vi "Reset Redlines.vi"(8 "error in (no error)":errorcluster, 11 "BluelinesRedlines in":refnum<class "BluelinesRedlines.lvclass">) -> (0 "error out":errorcluster, 3 "BluelinesRedlines out":refnum<class "BluelinesRedlines.lvclass">)   [LabVIEW 2020, in "VolatusGUIElements.lvlib" / "BluelinesRedlines.lvclass"]
uses:
  BluelinesRedlines.lvclass
  BluelinesRedlines.lvclass/BluelinesRedlines.ctl
  VolatusGUI/BluelinesRedlines Source/BluelinesRedlines Source.lvclass
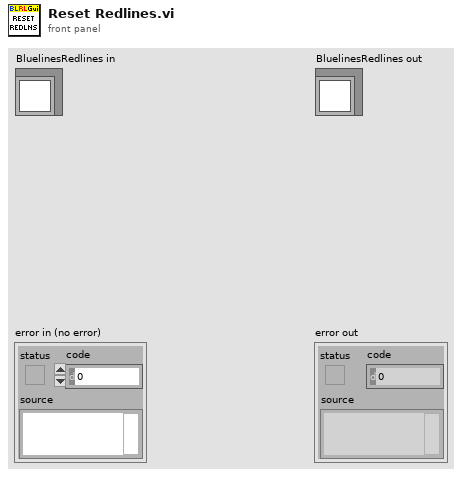
[diagram p1: front panel]
types:
  T1 = map{string, refnum<class "BluelinesRedlines Source.lvclass">}
  T2 = typedef "VolatusGUI.lvlib/BluelinesRedlines Source.lvclass/BLRL Config.ctl" = cluster{"Bluelines":T3[], "Redlines":T3[]}
  T3 = typedef "VolatusGUI.lvlib/BluelinesRedlines Source.lvclass/Range Limit Config.ctl" = cluster{"Channel":string, "Low Limit":dbl, "High Limit":dbl}
  T4 = typedef "VolatusGUIElements.lvlib/BluelinesRedlines.lvclass/Channel Info.ctl" = cluster{"Channel":refnum<class "Channel DBL.lvclass">, "Redline":bool}
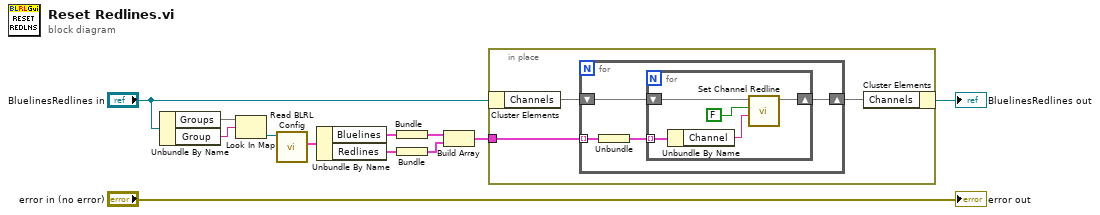
[diagram p0: block diagram]
diagram:
  n1 = Unbundle By Name("BluelinesRedlines in") -> ("Groups"=w4:T1, "Group"=w3:string)
  n2 = Look In Map(map=w4, key=w3) -> (value=w10:refnum<class "BluelinesRedlines Source.lvclass">)  [unwired: 1 in, 1 out]
  n3 = call-dynamic "Read BLRL Config.vi"("BluelinesRedlines Source in"=w10) -> ("BLRL Config"=w5:T2)  [unwired: 8 in, 2 out]
  n4 = Unbundle By Name(w5) -> ("Bluelines"=w9:T3[], "Redlines"=w8:T3[])
  n5 = Bundle("Bluelines"=w9) -> (w7:cluster{"Bluelines":T3[]})  [unwired: 1 in]
  n6 = Bundle("Redlines"=w8) -> (w6:cluster{"Redlines":T3[]})  [unwired: 1 in]
  n7 = Build Array(w7, w6) -> (w2:cluster{"Redlines":T3[]}[])
  n8 = in-place {
    in-place-border: w2 -> [w14]
    n9 = in-place-cluster #1("BluelinesRedlines in") -> ("Channels"=w15:map{string, T4})
    n10 = for {
      shift-right: [w17] -> w13
      shift-left: w15 -> [w18]
      tunnel: w14 -> [w19] mode=indexing
      n11 = Unbundle(w19) -> ("Redlines"=w16:T3[])
      n12 = for {
        shift-right: [w20] -> w17
        shift-left: w18 -> [w23]
        tunnel: w16 -> [w24] mode=indexing
        n13 = Unbundle By Name(w24) -> ("Channel"=w21:string)
        n14 = call "Set Channel Redline.vi"("Name"=w21, "Redline"=FALSE, "Channels in"=w23) -> ("Channels"=w20:map{string, T4})  [unwired: 7 in, 1 out]
      }
    }
    n15 = in-place-cluster #1("Channels"=w13) -> (→"BluelinesRedlines out":refnum<class "BluelinesRedlines.lvclass">)
  }
  "error out" <- "error in (no error)"
